vi "Add Interface Dialog.vi"(8 "error in":errorcluster, 11 "Target Item":T1) -> (0 "error out":errorcluster)   [LabVIEW 2020, in "Add Actor Interface.lvlib"]
uses:
  Add Actor Interface.lvlib
  AddActor/Support/Localized Strings.vi
  AddActor/Add Actor.lvlib
  MessageMakerProvider/AFPP Shared/AFPP Shared.lvlib
  <resource>/Framework/Providers/API/mxLvNIIM.ctl
panel:
  out "Path Display":string
  in  "Path":path caption="Save files to..."
  in  "Cancel Button":bool
  in  "OK Button":bool
  in  "Name of Interface":string
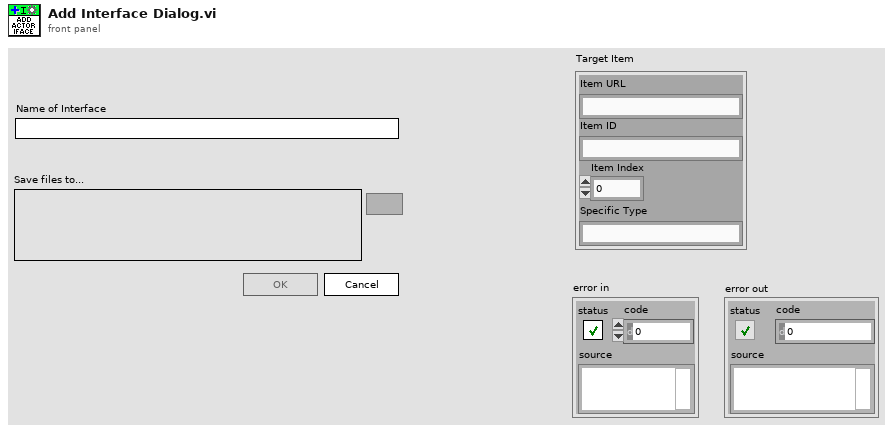
[diagram p1: front panel]
types:
  T1 = typedef "mxLvNIIM.ctl" = cluster{"Item URL":string, "Item ID":string, "Item Index":i32, "Specific Type":string}
  T2 = enum8{"Enabled", "Disabled", "Disabled and Grayed Out"}
  T3 = enum32{"Invalid", "Standard", "Closed", "Hidden", "Minimized", "Maximized"}
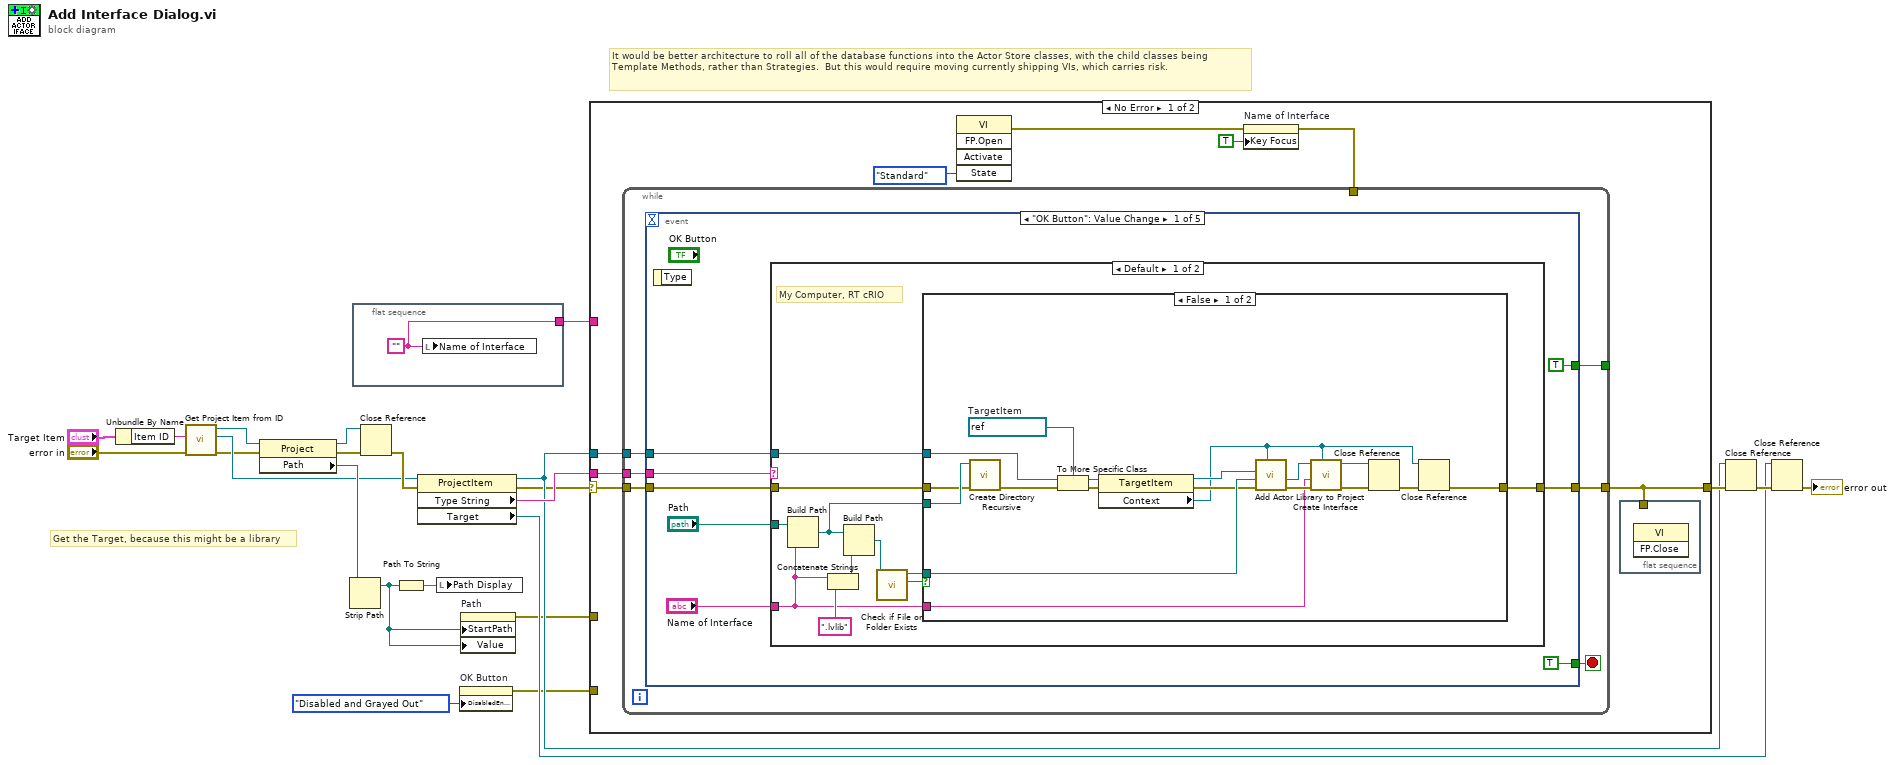
[diagram p0: block diagram]
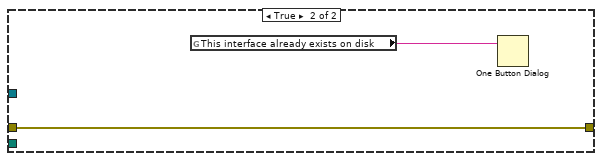
[diagram p2: hidden frame]
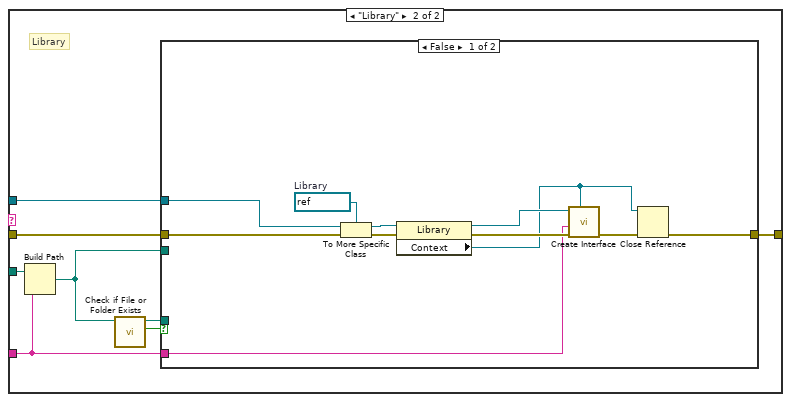
[diagram p3: hidden frame]
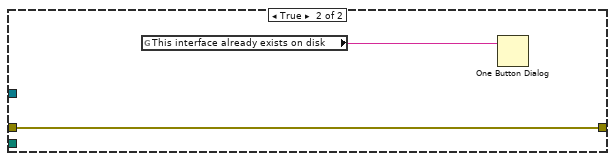
[diagram p4: hidden frame]
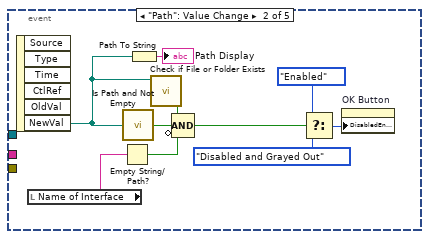
[diagram p5: hidden frame]
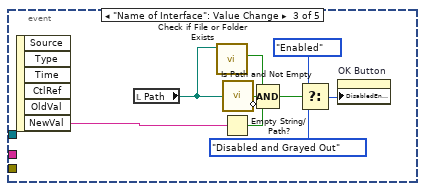
[diagram p6: hidden frame]
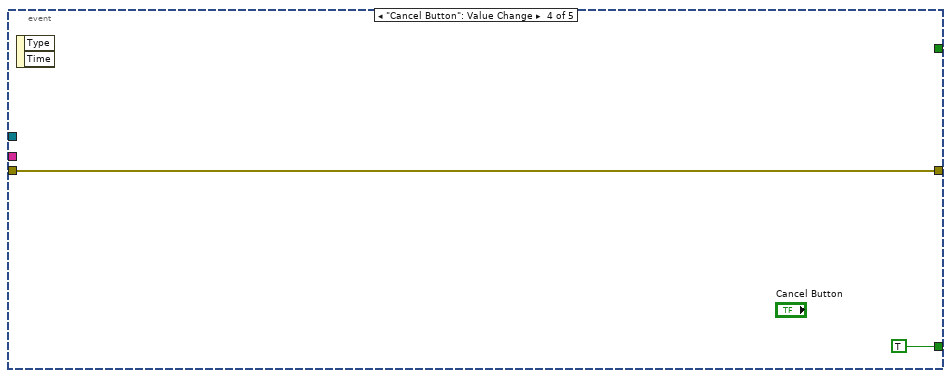
[diagram p7: hidden frame]
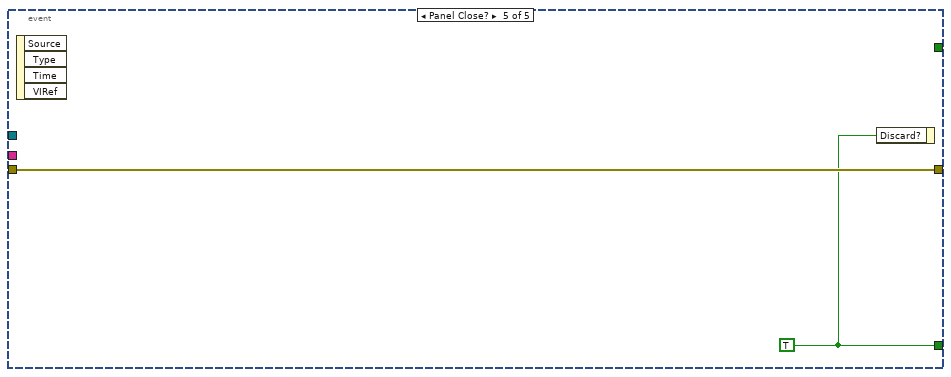
[diagram p8: hidden frame]
diagram:
  # "Get the Target, because this might be a library"
  # "It would be better architecture to roll all of the database functions into the Actor Store classes, with the child classes being Template Methods, rather than Strategies.  But this would require moving currently shipping VIs, which carries risk."
  n1 = Unbundle By Name("Target Item") -> ("Item ID"=w5:string)
  n2 = call "Get Project Item from ID.vi"("error in (no error)"="error in", "Item ID"=w5) -> ("error out"=w2:errorcluster, "Project Item"=w3:refnum<vi>, "Project out"=w4:refnum<vi>)  [unwired: 7 in]
  n3 = property class="Project"(reference=w4, error in=w2) -> (reference out=w15:refnum<vi>, error out=w17:errorcluster, "Path"=w22:path)
  n4 = Strip Path(path=w22) -> (stripped path=w18:path)  [unwired: 1 out]
  n5 = flat-sequence {
    tunnel: [w24] -> w9
    frame #0 {
      w24 = "" ("Name of Actor")
      n6 = local write "Name of Interface"(w24) -> ()
    }
  }
  n7 = Close Reference(reference=w15, error in (no error)=w17) -> (error out=w16:errorcluster)
  n8 = Path To String(path=w18) -> (string=w19:string)
  n9 = property class="ProjectItem"(reference=w3, error in=w16) -> (reference out=w11:refnum<vi>, error out=w8:errorcluster, "Type String"=w21:string, "Target"=w10:refnum<vi>)
  n10 = local write "Path Display"(w19) -> ()
  n11 = property on="OK Button" class="Bool"("DisabledEnum"=T2."Disabled and Grayed Out" ("Disabled")) -> (error out=w6:errorcluster)  [unwired: 2 in, 1 out]
  n12 = property on="Path" class="Path"("StartPath"=w18, "Value"=w18) -> (error out=w7:errorcluster)  [unwired: 2 in, 1 out]
  n13 = case shown="No Error" w8 {
    selector: w8 -> [w32 w122]
    tunnel: [w26 w122] -> w13
    tunnel: w21 -> [w31 _]
    tunnel: w11 -> [w30 _]
    tunnel: w9 -> [_ _]
    tunnel: w7 -> [_ _]
    tunnel: w6 -> [_ _]
    frame No Error {
      n14 = invoke class="VI" method="FP.Open"("State"=T3."Standard") -> (error out=w27:errorcluster)  [unwired: 4 in, 4 out]
      n15 = property on="Name of Interface" class="Str"(error in=w27, "Key Focus"=TRUE) -> (error out=w25:errorcluster)  [unwired: 1 in, 1 out]
      n16 = while {
        tunnel: [w38] -> w26
        tunnel: w32 -> [w37]
        tunnel: w31 -> [w35]
        tunnel: w30 -> [w34]
        tunnel: [w33] -> _
        tunnel: w25 -> [_]
        stop <- w36 stop-if-true
        n17 = event shown="[0] \"OK Button\": Value Change" {
          selector: _ -> [_ _ _ _ _]
          dyn-events: _ -> [_ _ _ _ _]
          timeout: _ -> [_ _ _ _ _]
          tunnel: w37 -> [w43 _ _ w118 w121]
          tunnel: [w44 _ _ w118 w121] -> w38
          tunnel: [TRUE _ _ TRUE w120] -> w36
          tunnel: w35 -> [w42 _ _ _ _]
          tunnel: w34 -> [w41 _ _ _ _]
          tunnel: [TRUE _ _ _ _] -> w33
          event "OK Button": Value Change {
            n18 = event-data() -> ()  [unwired: 1 in, 1 out]
            n19 = case shown="Default" w42 {
              tunnel: "Path" -> [w57 w85]
              tunnel: "Name of Interface" -> [w48 w79]
              tunnel: [w54 w83] -> w44
              tunnel: w43 -> [w53 w82]
              tunnel: w41 -> [w51 w80]
              frame Default {
                # "My Computer, RT cRIO"
                n20 = Build Path(base path=w57, name or relative path=w48) -> (appended path=w56:path)
                n21 = Concatenate Strings(w48, ".lvlib" ("string")) -> (w49:string)
                n22 = Build Path(base path=w56, name or relative path=w49) -> (appended path=w47:path)
                n23 = call <vilib>:"Check if File or Folder Exists.vi"("path"=w47) -> ("file or folder exists?"=w52:bool, "dup path"=w55:path)  [unwired: 8 in, 1 out]
                n24 = case shown="False" w52 {
                  tunnel: w48 -> [w68 _]
                  tunnel: w56 -> [w67 _]
                  tunnel: w55 -> [w75 _]
                  tunnel: [w59 w77] -> w54
                  tunnel: w53 -> [w66 w77]
                  tunnel: w51 -> [w69 _]
                  frame False {
                    w74 = refnum<vi> refnum  # TargetItem
                    n25 = call <vilib>:"Create Directory Recursive.vi"("error in (no error)"=w66, "directory"=w67) -> ("error out"=w65:errorcluster)  [unwired: 3 in, 2 out]
                    n26 = To More Specific Class(target class=w74, reference=w69, error in=w65) -> (specific class reference=w64:refnum<vi>, error out=w62:errorcluster)
                    n27 = property class="TargetItem"(reference=w64, error in=w62) -> (reference out=w63:refnum<vi>, error out=w61:errorcluster, "Context"=w58:refnum<vi>)
                    n28 = call "Add Actor Library to Project.vi"("Application"=w58, "error in (no error)"=w61, "Library Path"=w75, "Target Item"=w63) -> ("error out"=w73:errorcluster, "Library out"=w72:refnum<vi>)  [unwired: 6 in]
                    n29 = call "Create Interface.vi"("App Inst"=w58, "error in (no error)"=w73, "Actor Name"=w68, "Library in"=w72) -> ("error out"=w71:errorcluster, "Library out"=w70:refnum<vi>)  [unwired: 6 in]
                    n30 = Close Reference(reference=w70, error in (no error)=w71) -> (error out=w60:errorcluster)
                    n31 = Close Reference(reference=w58, error in (no error)=w60) -> (error out=w59:errorcluster)
                  }
                  frame True {
                    n32 = global read "Localized Strings.vi" "This interface already exists on disk"() -> (w76:string)
                    n33 = One Button Dialog(message=w76) -> ()  [unwired: 1 in, 1 out]
                  }
                }
              }
              frame "Library" {
                # "Library"
                n34 = Build Path(base path=w85, name or relative path=w79) -> (appended path=w78:path)
                n35 = call <vilib>:"Check if File or Folder Exists.vi"("path"=w78) -> ("file or folder exists?"=w81:bool, "dup path"=w84:path)  [unwired: 8 in, 1 out]
                n36 = case shown="False" w81 {
                  tunnel: w79 -> [w89 _]
                  tunnel: w78 -> [_ _]
                  tunnel: w84 -> [_ _]
                  tunnel: [w87 w98] -> w83
                  tunnel: w82 -> [w92 w98]
                  tunnel: w80 -> [w93 _]
                  frame False {
                    w96 = refnum<vi> refnum  # Library
                    n37 = To More Specific Class(target class=w96, reference=w93, error in=w92) -> (specific class reference=w95:refnum<vi>, error out=w94:errorcluster)
                    n38 = property class="Library"(reference=w95, error in=w94) -> (reference out=w91:refnum<vi>, error out=w90:errorcluster, "Context"=w86:refnum<vi>)
                    n39 = call "Create Interface.vi"("App Inst"=w86, "error in (no error)"=w90, "Actor Name"=w89, "Library in"=w91) -> ("error out"=w88:errorcluster)  [unwired: 6 in, 1 out]
                    n40 = Close Reference(reference=w86, error in (no error)=w88) -> (error out=w87:errorcluster)
                  }
                  frame True {
                    n41 = global read "Localized Strings.vi" "This interface already exists on disk"() -> (w97:string)
                    n42 = One Button Dialog(message=w97) -> ()  [unwired: 1 in, 1 out]
                  }
                }
              }
            }
          }
          event "Path": Value Change {
            n43 = event-data() -> ("NewVal"=w99:path)  [unwired: 1 in, 5 out]
            n44 = local read "Name of Interface"() -> (w105:string)
            n45 = Empty String/Path?(string/path=w105) -> (empty?=w104:bool)
            n46 = call <vilib>:"Is Path and Not Empty.vi"("path"=w99) -> ("Is Path and Not Empty?"=w103:bool)  [unwired: 4 in]
            n47 = Path To String(path=w99) -> (string=→"Path Display":string)
            n48 = call <vilib>:"Check if File or Folder Exists.vi"("path"=w99) -> ("file or folder exists?"=w100:bool)  [unwired: 8 in, 2 out]
            n49 = Compound Arithmetic op=AND(w100, w103, invert w104) -> (w102:bool)
            n50 = Select(t=T2."Enabled" ("Disabled"), s=w102, f=T2."Disabled and Grayed Out" ("Disabled")) -> (s? t:f=w107:T2)
            n51 = property on="OK Button" class="Bool"("DisabledEnum"=w107) -> ()  [unwired: 2 in, 2 out]
          }
          event "Name of Interface": Value Change {
            n52 = event-data() -> ("NewVal"=w111:string)  [unwired: 1 in, 5 out]
            n53 = local read "Path"() -> (w109:path)
            n54 = call <vilib>:"Check if File or Folder Exists.vi"("path"=w109) -> ("file or folder exists?"=w110:bool)  [unwired: 8 in, 2 out]
            n55 = Empty String/Path?(string/path=w111) -> (empty?=w114:bool)
            n56 = call <vilib>:"Is Path and Not Empty.vi"("path"=w109) -> ("Is Path and Not Empty?"=w113:bool)  [unwired: 4 in]
            n57 = Compound Arithmetic op=AND(w110, w113, invert w114) -> (w112:bool)
            n58 = Select(t=T2."Enabled" ("Disabled"), s=w112, f=T2."Disabled and Grayed Out" ("Disabled")) -> (s? t:f=w116:T2)
            n59 = property on="OK Button" class="Bool"("DisabledEnum"=w116) -> ()  [unwired: 2 in, 2 out]
          }
          event "Cancel Button": Value Change {
            n60 = event-data() -> ()  [unwired: 1 in, 2 out]
          }
          event Panel Close? {
            w120 = TRUE
            n61 = event-data() -> ()  [unwired: 1 in, 4 out]
            n62 = event-data("Discard?"=w120) -> ()  [unwired: 1 in, 1 out]
          }
        }
      }
      n63 = flat-sequence {
        tunnel: w26 -> [_]
        frame #0 {
          n64 = invoke class="VI" method="FP.Close"() -> ()  [unwired: 3 in, 3 out]
        }
      }
    }
    frame Error {
    }
  }
  n65 = Close Reference(reference=w11, error in (no error)=w13) -> (error out=w14:errorcluster)
  n66 = Close Reference(reference=w10, error in (no error)=w14) -> (error out=→"error out":errorcluster)
